vi "From Serial Form.vi"(6 "Serial Version":T1, 10 "Deserializer in":refnum<class "Deserializer.lvclass">, 11 "Humidity Control in":refnum<class "Humidity Control.lvclass">) -> (0 "error out":errorcluster, 2 "Deserializer out":refnum<class "Deserializer.lvclass">, 3 "Humidity Control out":refnum<class "Humidity Control.lvclass">)   [LabVIEW 2012, in "Humidity Control.lvclass"]
uses:
  Humidity Control.lvclass
  <userlib>/Serialization/Serializable/Serializable.lvclass
  <userlib>/Serialization/Serializable/Remove Single.vi
  <userlib>/Serialization/Serializable/Remove Double.vi
  <userlib>/Serialization/Serialization Common/Serial Version.ctl
  <userlib>/Serialization/Serialization Common/Serialization Common.lvlib
  <userlib>/Serialization/Deserializer/Deserializer.lvclass
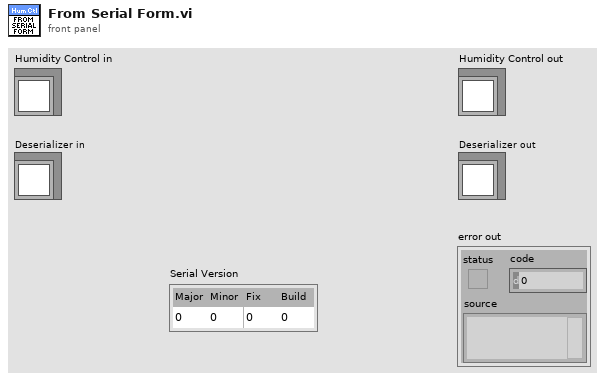
[diagram p1: front panel]
types:
  T1 = typedef "Serialization Common.lvlib/Serial Version.ctl" = cluster{"Major":u16, "Minor":u16, "Fix":u16, "Build":u16}
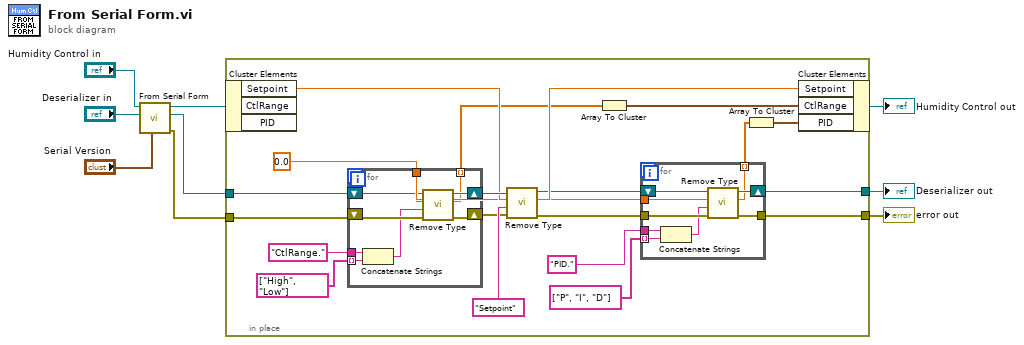
[diagram p0: block diagram]
diagram:
  n1 = call-parent "From Serial Form.vi"("Serial Version"="Serial Version", "Deserializer in"="Deserializer in", "Serializable in"="Humidity Control in") -> ("error out"=w4:errorcluster, "Deserializer out"=w5:refnum<class "Deserializer.lvclass">, "Serializable out"=w6:refnum<class "Humidity Control.lvclass">)  [unwired: 6 in]
  n2 = in-place {
    in-place-border: w5 -> [w29]
    in-place-border: w4 -> [w28]
    in-place-border: [w21] -> w3
    in-place-border: [w11] -> w1
    w15 = 0.0
    n3 = in-place-cluster #1(w6) -> ("Setpoint"=w26:sgl)  [unwired: 2 out]
    n4 = for {
      shift-right: [w45] -> w27
      shift-left: w29 -> [w47]
      shift-right: [w40] -> w18
      shift-left: w28 -> [w46]
      tunnel: w15 -> [w44]
      tunnel: string[] ["High", "Low"] -> [w43] mode=indexing
      tunnel: "CtlRange." ("Name") -> [w42]
      tunnel: [w39] -> w17 mode=indexing
      n5 = Concatenate Strings(w42, w43) -> (w41:string)
      n6 = call-poly <userlib>:"Remove Type.vi"("error in (no error)"=w46, "Name"=w41, "Default Value"=w44, "Deserializer in"=w47) -> ("error out"=w40:errorcluster, "Numeric"=w39:dbl, "Deserializer out"=w45:refnum<class "Deserializer.lvclass">)  [unwired: 4 in, 1 out]
    }
    n7 = call-poly <userlib>:"Remove Type.vi"("error in (no error)"=w18, "Name"="Setpoint", "Default Value"=w26, "Deserializer in"=w27) -> ("error out"=w22:errorcluster, "Numeric"=w25:sgl, "Deserializer out"=w23:refnum<class "Deserializer.lvclass">)  [unwired: 4 in, 1 out]
    n8 = Array To Cluster(array=w17) -> (cluster=w16:cluster{"[0]":dbl, "[1]":dbl})
    n9 = for {
      tunnel: w22 -> [w37]
      tunnel: w15 -> [w35]
      tunnel: string[] ["P", "I", "D"] -> [w34] mode=indexing
      tunnel: "PID." ("Name") -> [w33]
      tunnel: [w31] -> w12 mode=indexing
      shift-right: [w36] -> w21
      shift-left: w23 -> [w38]
      tunnel: [w30] -> w11
      n10 = Concatenate Strings(w33, w34) -> (w32:string)
      n11 = call-poly <userlib>:"Remove Type.vi"("error in (no error)"=w37, "Name"=w32, "Default Value"=w35, "Deserializer in"=w38) -> ("error out"=w30:errorcluster, "Numeric"=w31:dbl, "Deserializer out"=w36:refnum<class "Deserializer.lvclass">)  [unwired: 4 in, 1 out]
    }
    n12 = Array To Cluster(array=w12) -> (cluster=w10:cluster{"[0]":dbl, "[1]":dbl, "[2]":dbl})
    n13 = in-place-cluster #1("Setpoint"=w25, "CtlRange"=w16, "PID"=w10) -> (→"Humidity Control out":refnum<class "Humidity Control.lvclass">)
  }
  "error out" <- w1
  "Deserializer out" <- w3
